vi "Sub_filename.vi"(8 "Window":i32, 9 "Particles":i32, 10 "Nodes":i32, 11 "Method":i32) -> (3 "Filename":string)   [LabVIEW 2019]
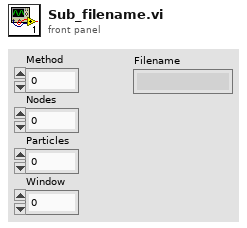
[diagram p1: front panel]
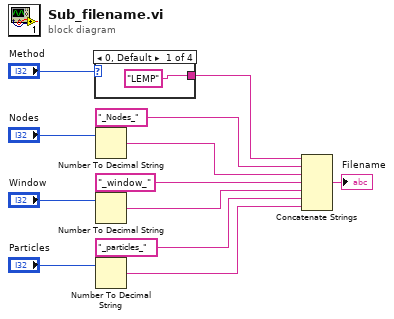
[diagram p0: block diagram]
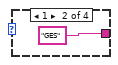
[diagram p2: hidden frame]
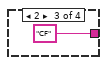
[diagram p3: hidden frame]
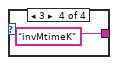
[diagram p4: hidden frame]
diagram:
  n1 = case shown="0, Default" "Method" {
    tunnel: ["LEMP" "GES" "CF" "invMtimeK"] -> w8
    frame 0, Default {
    }
    frame 1 {
    }
    frame 2 {
    }
    frame 3 {
    }
  }
  n2 = Number To Decimal String(number="Nodes") -> (decimal integer string=w6:string)  [unwired: 1 in]
  n3 = Number To Decimal String(number="Window") -> (decimal integer string=w4:string)  [unwired: 1 in]
  n4 = Number To Decimal String(number="Particles") -> (decimal integer string=w2:string)  [unwired: 1 in]
  n5 = Concatenate Strings(w8, "_Nodes_", w6, "_window_", w4, "_particles_", w2) -> (→"Filename":string)
